vi "Get Variables.vi"(8 "error in (no error)":errorcluster, 11 "For Loop in":refnum<class "Structure If Else.lvclass">) -> (0 "error out":errorcluster, 2 "Variables":variant, 3 "For Loop out":refnum<class "Structure If Else.lvclass">)   [LabVIEW 2016, in "Structure If Else.lvclass"]
uses:
  Structure If Else.lvclass
  Structure If Else.lvclass/Structure If Else.ctl
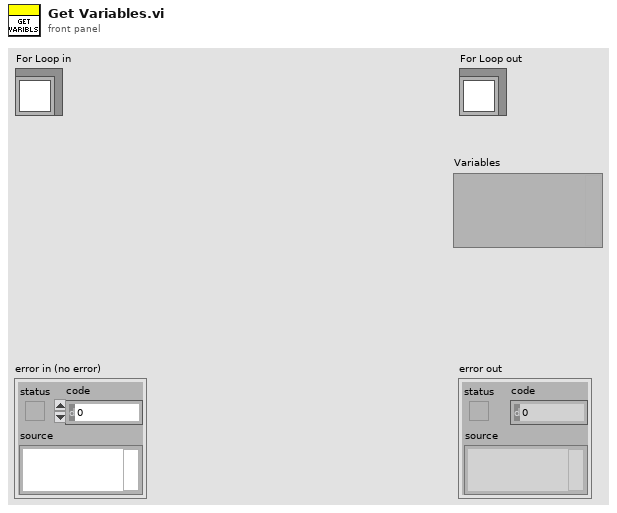
[diagram p1: front panel]
types:
  T1 = typedef "Structure If Else.lvclass/Variables.ctl" = cluster{"Start":dbl, "Stop":dbl, "Step":dbl}
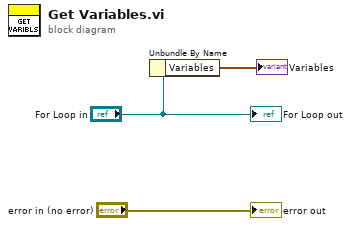
[diagram p0: block diagram]
diagram:
  n1 = Unbundle By Name("For Loop in") -> ("Variables"=→"Variables":T1)
  "error out" <- "error in (no error)"
  "For Loop out" <- "For Loop in"
